vi "Add Analyzer.vi"(8 "error in (no error)":errorcluster, 10 "new plugin":refnum<class "Generic Plugin.lvclass">, 11 "Plugin Array in":refnum<class "Controller Array.lvclass">) -> (0 "error out":errorcluster, 3 "Plugin Array out":refnum<class "Controller Array.lvclass">)   [LabVIEW 2020, in "RxnRover.lvlib"]
doc: "Adds a new analyzer plugin to the process cache."
uses:
  RxnRover.lvlib
  Controller Array/Controller Array.lvclass
  Controller/Generic Plugin.lvclass
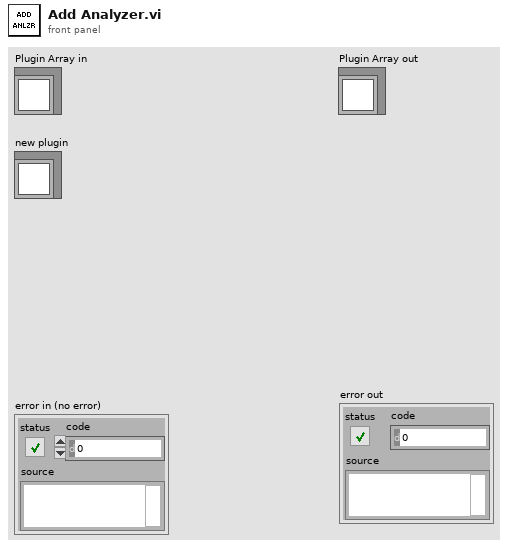
[diagram p1: front panel]
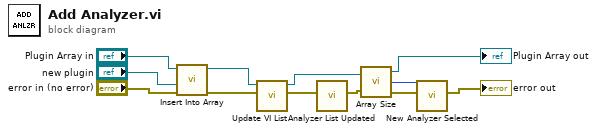
[diagram p0: block diagram]
diagram:
  n1 = call "Insert Into Array.vi"("error in (no error)"="error in (no error)", "new element"="new plugin", "Controller Array in"="Plugin Array in") -> ("error out"=w4:errorcluster, "Controller Array out"=w2:refnum<class "Controller Array.lvclass">)  [unwired: 2 in, 1 out]
  n2 = call "Update VI List.vi"("error in (no error)"=w4, "Controller Array in"=w2) -> ("error out"=w3:errorcluster, "Controller Array out"=w1:refnum<class "Controller Array.lvclass">)  [unwired: 8 in]
  n3 = call "Analyzer List Updated.vi"("error in (no error)"=w3) -> ("error out"=w9:errorcluster)  [unwired: 10 in]
  n4 = call "Array Size.vi"("Controller Array in"=w1, "error in (no error)"=w9) -> ("Controller Array out"=→"Plugin Array out":refnum<class "Controller Array.lvclass">, "size(s)"=w7:i32, "error out"=w8:errorcluster)
  n5 = call "New Analyzer Selected.vi"("error in (no error)"=w8, "Analyzer Index"=w7) -> ("error out"=→"error out":errorcluster)  [unwired: 9 in]
